vi "FT 1 (2).vi"() -> ()   [LabVIEW 2020]
uses:
  <vilib>/addons/Control Design/_Model Construction/Model Creation.llb/Model Creation SubVI/cd_Create State Space Model.vi
  <vilib>/addons/Control Design/_Utility/Model Viewer.llb/Model Viewer SubVI/cd_Draw Zero-Pole-Gain Equation (SS).vi
  <vilib>/addons/Control Design/_Utility/Model Viewer.llb/Model Viewer SubVI/cd_Draw Transfer Function Equation (SS).vi
  <vilib>/imath/engines/lvmath2/RunTimeSupport/NIMS_Get Any Vector_w Error - Matrix.vi
  <instcachedir>/0/NIMS_Get Any Vector_w Error - Matrix_03E716A238FA4CA1B10D931DADE97109.lvgen/NIMS_Get Any Vector_w Error - Matrix_03E716A238FA4CA1B10D931DADE97109_001.vi
  <vilib>/imath/engines/lvmath2/RunTimeSupport/NIMS_Get Scalar_w Error.vi
  <instcachedir>/0/NIMS_Get Scalar_w Error_5A0E401CB6154DCF81784DB8E431B6E1.lvgen/NIMS_Get Scalar_w Error_5A0E401CB6154DCF81784DB8E431B6E1_010.vi
  <vilib>/imath/engines/lvmath2/RunTimeEngine/BuiltInFunctions/ss_to_tf/NIMS_ss_to_tf(4i).vi
  <vilib>/imath/engines/lvmath2/RunTimeEngine/ErrorHandling/NIMS_Create Error From Enums.vi
  <vilib>/imath/engines/lvmath/Plug In/Control Design/BuiltInFunctions/tf/NIMS_CD_tf(num,den,Ts).vi
  <vilib>/imath/engines/lvmath/Plug In/Control Design/BuiltInFunctions/ackermann/NIMS_CD_ackermann(A,B,poles,STR).vi
  <vilib>/imath/engines/lvmath2/RunTimeEngine/ArithmeticOperatorToken/NIMS_ArithmeticOperator_multmx.vi
  <instcachedir>/0/NIMS_ArithmeticOperator_multmx_177F0753FB7A49B190E35F5DD0E80316.lvgen/NIMS_ArithmeticOperator_multmx_177F0753FB7A49B190E35F5DD0E80316_004.vi
  <vilib>/imath/engines/lvmath2/RunTimeEngine/ArithmeticOperatorToken/NIMS_ArithmeticOperator_minus.vi
  <instcachedir>/0/NIMS_ArithmeticOperator_minus_822089A08BE049DB927E6BEA78E100F1.lvgen/NIMS_ArithmeticOperator_minus_822089A08BE049DB927E6BEA78E100F1_002.vi
  <vilib>/imathl/engines/lvmath/Functions/Error Handling/Create Error.vi
  <vilib>/imath/engines/lvmath2/RunTimeEngine/NodeEndStatement/NIMS_NodeEndStatement_Output.vi
  <instcachedir>/0/NIMS_NodeEndStatement_Output_53EC0D466D134D7ABD903AC30B43404B.lvgen/NIMS_NodeEndStatement_Output_53EC0D466D134D7ABD903AC30B43404B_010.vi
  <instcachedir>/0/NIMS_NodeEndStatement_Output_53EC0D466D134D7ABD903AC30B43404B.lvgen/NIMS_NodeEndStatement_Output_53EC0D466D134D7ABD903AC30B43404B_005.vi
  <vilib>/imath/engines/lvmath2/RunTimeEngine/ErrorHandling/NIMS_Finalize Error.vi
  <vilib>/addons/Control Design/_Utility/Model Viewer.llb/Model Viewer SubVI/cd_Draw Transfer Function Equation (TF).vi
  <vilib>/addons/Control Design/_Time Response Analysis/Time Response.llb/Time Response subVI/cd_Step Response (Transfer Function).vi
  <vilib>/addons/Control Design/_Utility/Model Viewer.llb/Model Viewer SubVI/cd_Draw Zero-Pole-Gain Equation (TF).vi
  <vilib>/addons/Control Design/_Model Construction/NI_LinSys_Model Creation.lvlib
  <vilib>/addons/Control Design/_Utility/NI_CD_Model Viewer.lvlib
  <vilib>/addons/Control Design/_Time Response Analysis/NI_CD_Time Response.lvlib
panel:
  out "Plnta 2":picture
  out "Equation 6":picture
  out "Step Response Graph 4":cluster{"time":dbl[], dbl[]}[](graph)
  out "Equation 5":picture
  out "Ke":dbl[](array[numeric])
  out "Step Response Graph 3":cluster{"time":dbl[], dbl[]}[](graph)
  out "Step Response Graph 2":cluster{"time":dbl[], dbl[]}[](graph)
  out "Step Response Graph":cluster{"time":dbl[], dbl[]}[](graph)
  out "Equation 4":picture
  out "Equation 3":picture
  out "K":dbl[](array[numeric])
  out "Equation 2":picture
  out "Planta 1":picture
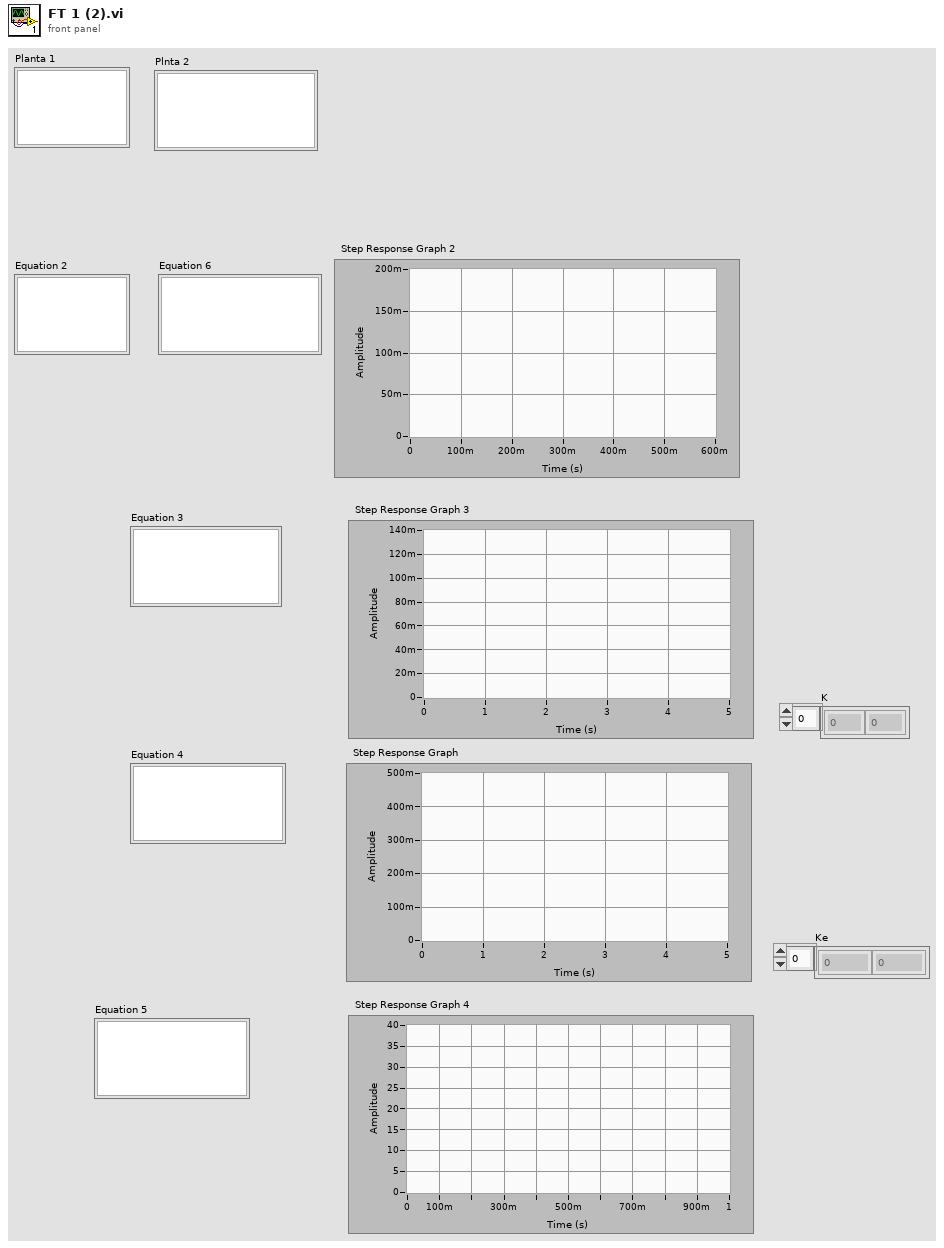
[diagram p1: front panel]
types:
  T1 = typedef "NI_LinSys_Model Typedefs.lvlib/CD Transfer Function Model (MIMO).ctl" = cluster{"properties":T2, "transfer function(s)":T3[][]}
  T2 = typedef "NI_LinSys_Model Typedefs.lvlib/CD General Elements.ctl" = cluster{"Model name":string, "Input names":string[], "Output names":string[], "Input Delays":dbl[], "Output Delays":dbl[], "Sampling Time":dbl, "Notes":string}
  T3 = typedef "NI_LinSys_Model Typedefs.lvlib/CD Transfer Function Model (SISO).ctl" = cluster{"Numerator":dbl[], "Denominator":dbl[], "delay":dbl}
  T4 = typedef "NI_LinSys_Model Typedefs.lvlib/CD State Space Model (MIMO).ctl" = cluster{"properties":T2, "A":dbl[][], "B":dbl[][], "C":dbl[][], "D":dbl[][], "StateNames":string[], "Transport Delay":dbl[][]}
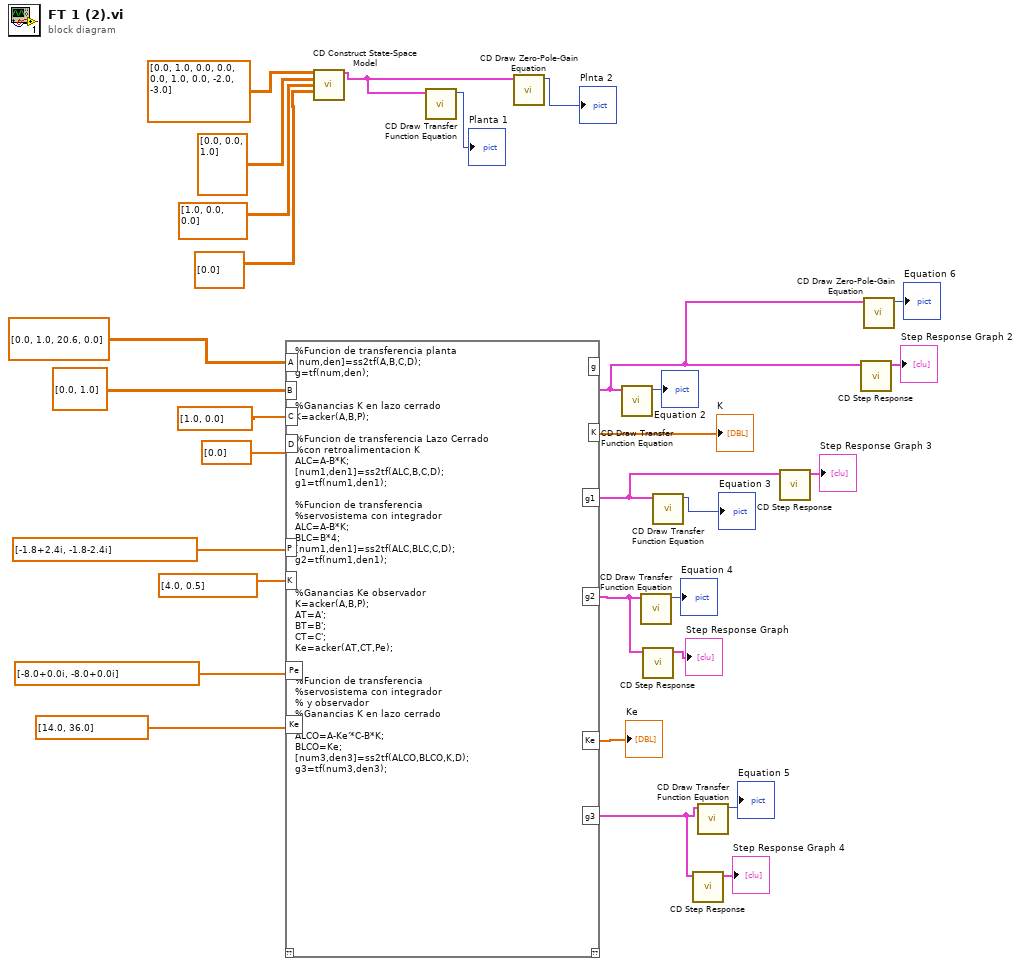
[diagram p0: block diagram]
diagram:
  n1 = mathscript code="%Funcion de transferencia planta\n[num,den]=ss2tf(A,B,C,D);\ng=tf(num,den);\n\n\n%Ganancias K en lazo cerrado\nK=acker(A,B,P);\n\n%Funcion de transferencia Lazo Cerrado\n%con retroalimentacion K\nALC=A-B*K;\n[num1,den1]=ss2tf(ALC,B,C,D);\ng1=tf(num1,den1);\n\n%Funcion de transferencia \n%servosistema con integrador\nALC=A-B*K;\nBLC=B*4;\n[num1,den1]=ss2tf(ALC,BLC,C,D);\ng2=tf(num1,den1);\n\n\n%Ganancias Ke observador\nK=acker(A,B,P);\nAT=A';\nBT=B';\nCT=C';\nKe=acker(AT,CT,Pe);\n\n\n%Funcion de transferencia \n%servosistema con integrador\n% y observador\n%Ganancias K en lazo cerrado\n\nALCO=A-Ke'*C-B*K;\nBLCO=Ke;\n[num3,den3]=ss2tf(ALCO,BLCO,K,D);\ng3=tf(num3,den3);"("A"=dbl[][] [[0.0, 1.0], [20.6, 0.0]], "B"=dbl[][] [[0.0], [1.0]], "C"=dbl[] [1.0, 0.0], "D"=dbl[] [0.0], "P"=cdb[] [-1.8+2.4i, -1.8-2.4i] ("Polos Propuestos"), "K"=dbl[] [4.0, 0.5] ("K1 2"), "Pe"=cdb[] [-8.0+0.0i, -8.0+0.0i] ("Polos Propuestos"), "Ke"=dbl[] [14.0, 36.0] ("K1 2")) -> ("g"=w2:T1, "K"=→"K":dbl[], "g1"=w11:T1, "g2"=w15:T1, "Ke"=→"Ke":dbl[], "g3"=w1:T1)  [unwired: 1 in, 1 out]
  n2 = call-poly <vilib>:"CD Construct State-Space Model.vi"("A"=dbl[][] [[0.0, 1.0, 0.0], [0.0, 0.0, 1.0], [0.0, -2.0, -3.0]], "B"=dbl[][] [[0.0], [0.0], [1.0]], "C"=dbl[][] [[1.0, 0.0, 0.0]], "D"=dbl[][] [[0.0]]) -> ("State-Space Model"=w3:T4)  [unwired: 10 in, 1 out]
  n3 = call-poly <vilib>:"CD Draw Transfer Function Equation.vi"("State-Space Model"=w3) -> ("Equation"=→"Planta 1":picture)  [unwired: 8 in, 2 out]
  n4 = call-poly <vilib>:"CD Draw Zero-Pole-Gain Equation.vi"("State-Space Model"=w3) -> ("Equation"=→"Plnta 2":picture)  [unwired: 8 in, 2 out]
  n5 = call-poly <vilib>:"CD Draw Transfer Function Equation.vi"("Transfer Function Model"=w2) -> ("Equation"=→"Equation 2":picture)  [unwired: 8 in, 2 out]
  n6 = call-poly <vilib>:"CD Draw Transfer Function Equation.vi"("Transfer Function Model"=w15) -> ("Equation"=→"Equation 4":picture)  [unwired: 8 in, 2 out]
  n7 = call-poly <vilib>:"CD Step Response.vi"("Transfer Function Model"=w15) -> ("Step Response Graph"=→"Step Response Graph":cluster{"time":dbl[], dbl[]}[])  [unwired: 8 in, 2 out]
  n8 = call-poly <vilib>:"CD Draw Transfer Function Equation.vi"("Transfer Function Model"=w11) -> ("Equation"=→"Equation 3":picture)  [unwired: 8 in, 2 out]
  n9 = call-poly <vilib>:"CD Step Response.vi"("Transfer Function Model"=w1) -> ("Step Response Graph"=→"Step Response Graph 4":cluster{"time":dbl[], dbl[]}[])  [unwired: 8 in, 2 out]
  n10 = call-poly <vilib>:"CD Draw Transfer Function Equation.vi"("Transfer Function Model"=w1) -> ("Equation"=→"Equation 5":picture)  [unwired: 8 in, 2 out]
  n11 = call-poly <vilib>:"CD Step Response.vi"("Transfer Function Model"=w11) -> ("Step Response Graph"=→"Step Response Graph 3":cluster{"time":dbl[], dbl[]}[])  [unwired: 8 in, 2 out]
  n12 = call-poly <vilib>:"CD Step Response.vi"("Transfer Function Model"=w2) -> ("Step Response Graph"=→"Step Response Graph 2":cluster{"time":dbl[], dbl[]}[])  [unwired: 8 in, 2 out]
  n13 = call-poly <vilib>:"CD Draw Zero-Pole-Gain Equation.vi"("Transfer Function Model"=w2) -> ("Equation"=→"Equation 6":picture)  [unwired: 8 in, 2 out]
